vi "Discard correct num element.vi"(8 "Read packet dim":i32, 11 "Element Remaing in Queue":i32) -> (3 "Effective read element":i32)   [LabVIEW 2014]
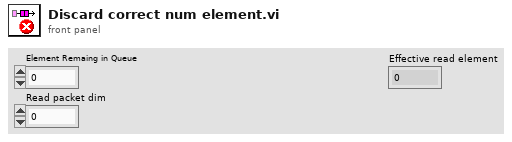
[diagram p1: front panel]
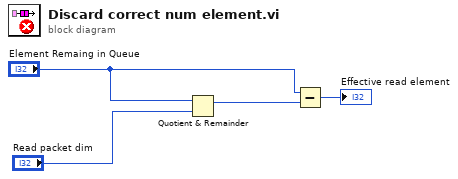
[diagram p0: block diagram]
diagram:
  n1 = Quotient & Remainder(x="Element Remaing in Queue", y="Read packet dim") -> (x-y*floor(x/y)=w2:i32)  [unwired: 1 out]
  n2 = Subtract(x="Element Remaing in Queue", y=w2) -> (x-y=→"Effective read element":i32)
